vi "Voltage_Input_Super.vi"() -> ()   [LabVIEW 2018]
doc: "This example demonstrates how to continuously acquire buffered voltage measurements using a DAQmx device.\n\nFor instructions on how to connect your signals to the DAQ device, refer to your device documentation."
uses:
  <vilib>/Utility/error.llb/DialogType.ctl
  <vilib>/DAQmx/read.llb/DAQmx Read (Analog 1D Wfm NChan NSamp).vi
  <vilib>/DAQmx/create/channels.llb/DAQmx Create Channel (AI-Voltage-Basic).vi
  <vilib>/DAQmx/configure/timing.llb/DAQmx Timing (Sample Clock).vi
  <vilib>/DAQmx/miscellaneous.llb/DAQmx Fill In Error Info.vi
  <resource>/objmgr/daqmx.rc
panel:
  in  "index":i32
  out "Waveform Chart 5":waveform(dbl)(graph)
  out "Waveform Chart 4":waveform(dbl)[](graph)
  in  "Channel":i32
  in  "Channel":i32
  out "Waveform Chart 3":waveform(dbl)(graph)
  in  "samples per channel":i32=1000
  in  "Stop 2":bool
  out "Waveform Chart 2":waveform(dbl)(graph)
  in  "name or relative path":string
  in  "Sample Rate":dbl=1000.0
  in  "Max Voltage":dbl=5.0
  in  "Min Voltage":dbl=-5.0
  in  "Physical Channel":tag="Dev1/ai0"
  out "Actual Sample Rate":dbl=1000.0 format="%0.2f"
  # "Volt Input"
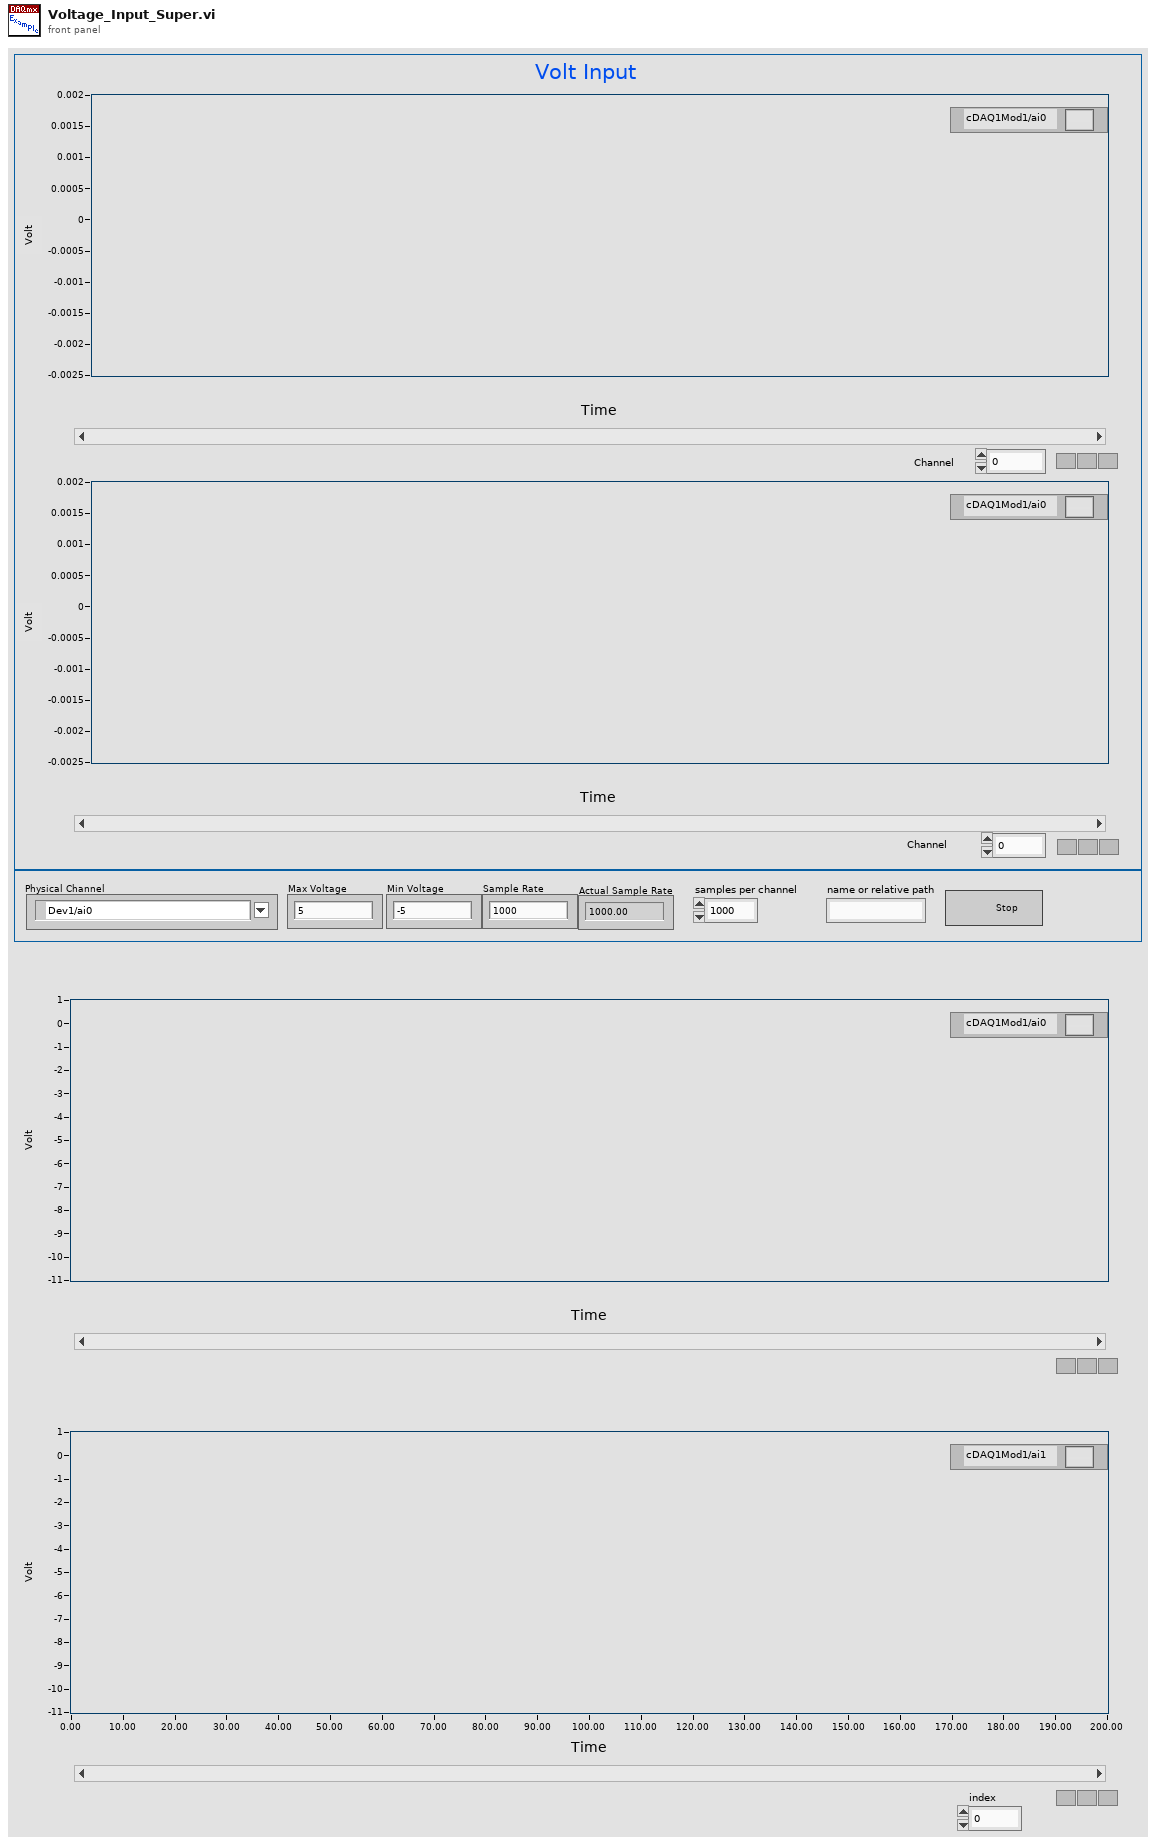
[diagram p1: front panel]
types:
  T1 = typedef "DialogType.ctl" = u16
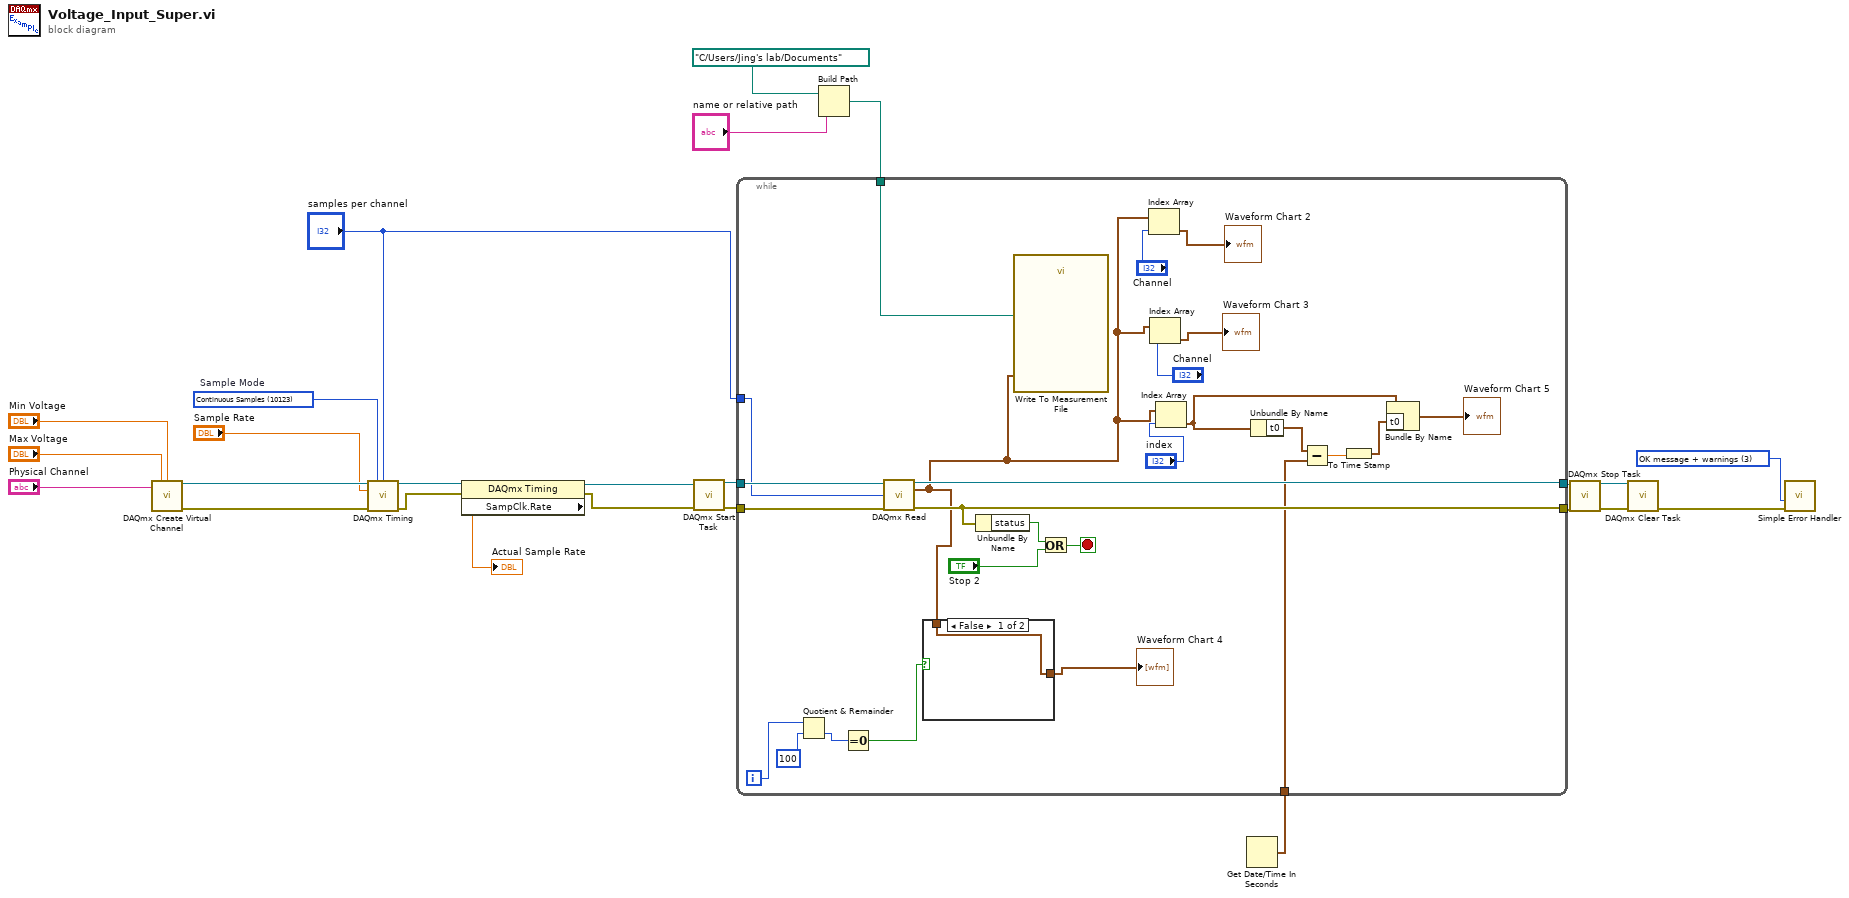
[diagram p0: block diagram]
diagram:
  w8 = T1 3 items=["no dialog", "OK message", "continue or stop message", "OK message + warnings", "continue/stop + warnings"] ("type of dialog (OK msg:1)")
  w23 = 10123 items=["Finite Samples"=10178, "Continuous Samples"=10123, "Hardware Timed Single Point"=12522]  # Sample Mode
  n1 = call-poly <vilib>:"DAQmx Create Virtual Channel.vi"("maximum value"="Max Voltage", "minimum value"="Min Voltage", "physical channels"="Physical Channel") -> ("task out"=w21:refnum<k21>, "error out"=w22:errorcluster)  [unwired: 11 in]
  n2 = call-poly <vilib>:"DAQmx Timing.vi"("task/channels in"=w21, "sample mode"=w23, "samples per channel"="samples per channel", "rate"="Sample Rate", "error in"=w22) -> ("task out"=w25:refnum<k21>, "error out"=w24:errorcluster)  [unwired: 9 in]
  n3 = property class="DAQmx Timing"(reference=w25, error in=w24) -> (reference out=w4:refnum<k21>, error out=w5:errorcluster, "SampClk.Rate"=→"Actual Sample Rate":dbl)
  n4 = call <vilib>:"DAQmx Start Task.vi"("task/channels in"=w4, "error in"=w5) -> ("task out"=w20:refnum<k21>, "error out"=w19:errorcluster)  [unwired: 12 in]
  n5 = Build Path(base path=path "C:/Users/Jing's lab/Documents", name or relative path="name or relative path") -> (appended path=w3:path)
  n6 = Get Date/Time In Seconds() -> (seconds since 1Jan1904=w1:timestamp)
  n7 = while {
    tunnel: w20 -> [w51]
    tunnel: w19 -> [w50]
    tunnel: [w49] -> w12
    tunnel: [w48] -> w11
    tunnel: w3 -> [w45]
    tunnel: "samples per channel" -> [w43]
    tunnel: w1 -> [w31]
    i -> [w36]
    stop <- w46 stop-if-true
    n8 = Quotient & Remainder(x=w36, y=100) -> (floor(x/y)=w38:i32)  [unwired: 1 out]
    n9 = Equal To 0?(x=w38) -> (x = 0?=w35:bool)
    n10 = call-poly <vilib>:"DAQmx Read.vi"("task/channels in"=w51, "number of samples per channel"=w43, "error in"=w50) -> ("task out"=w49:refnum<k21>, "data"=w33:waveform(dbl)[], "error out"=w48:errorcluster)  [unwired: 10 in]
    n11 = case shown="False" w35 {
      tunnel: [w52 w53] -> w34
      tunnel: w33 -> [w52 w53]
      frame False {
      }
      frame True {
      }
    }
    "Waveform Chart 4" <- w34
    n12 = Unbundle By Name(w48) -> ("status"=w47:bool)
    n13 = call "Write To Measurement File"("Signals"=w33, "Filename"=w45) -> ()  [unwired: 15 in, 3 out]
    n14 = Or(x=w47, y="Stop 2") -> (x .or. y?=w46:bool)
    n15 = Index Array(array=w33, index="Channel") -> (element=→"Waveform Chart 2":waveform(dbl))
    n16 = Index Array(array=w33, index="Channel") -> (element=→"Waveform Chart 3":waveform(dbl))
    n17 = Index Array(array=w33, index="index") -> (element=w28:waveform(dbl))
    n18 = Unbundle By Name(w28) -> ("t0"=w32:timestamp)
    n19 = Subtract(x=w32, y=w31) -> (x-y=w30:dbl)
    n20 = To Time Stamp(1:w30) -> (0:w29:timestamp)
    n21 = Bundle By Name(cluster=w28, "t0"=w29) -> (→"Waveform Chart 5":waveform(dbl))
  }
  n22 = call <vilib>:"DAQmx Stop Task.vi"("task/channels in"=w12, "error in"=w11) -> ("task out"=w9:refnum<k21>, "error out"=w10:errorcluster)  [unwired: 12 in]
  n23 = call <vilib>:"DAQmx Clear Task.vi"("task in"=w9, "error in"=w10) -> ("error out"=w18:errorcluster)  [unwired: 13 in]
  n24 = call <vilib>:"Simple Error Handler.vi"("type of dialog (OK msg:1)"=w8, "error in (no error)"=w18) -> ()  [unwired: 3 in, 5 out]
